vi "运维调试_五参数.vi"(11 "编号":string) -> ()   [LabVIEW 2016, in "斯坦道多参数.lvlib"]
uses:
  <vilib>/Utility/miscctls.llb/LVPointTypeDef.ctl
  <vilib>/Plasmionique/MB Master/MB_Master/MB_Master.lvclass
  <vilib>/ptbypt/NI_PtbyPt.lvlib
  <vilib>/Utility/config.llb/NI_LVConfig.lvlib
panel:
  in  "Serial Config":T1={"baud rate (bps)"=9600, "stop bits"=10, "parity"=0, "flow control"=0, "timeout"=2000, "retries"=1} {"stop bits" items=["1.0"=10, "1.5"=15, "2.0"=20]; "parity" items=["None", "Odd", "Even", "Mark", "Space"]; "flow control" items=["None", "XON/XOFF", "RTS/CTS", "XON/XOFF & RTS/CTS", "DTR/DSR", "XON/XOFF & DTR/DSR"]}
  in  "探头设置":bool
  in  "量程设置":bool
  out "显示框":T2={"显示控件"={"标题背景颜色"=3381759, "监测值背景颜色"=16777226, "监测参数"="", "状态1"="", "状态2"="", "数据标识"=""}, "显示控件 2"={"标题背景颜色"=3381759, "监测值背景颜色"=16777226, "监测参数"="", "状态1"="", "状态2"="", "数据标识"=""}, "显示控件 3"={"标题背景颜色"=3381759, "监测值背景颜色"=16777226, "监测参数"="", "状态1"="", "状态2"="", "数据标识"=""}, "显示控件 4"={"标题背景颜色"=3381759, "监测值背景颜色"=16777226, "监测参数"="", "状态1"="", "状态2"="", "数据标识"=""}, "显示控件 5"={"标题背景颜色"=3381759, "监测值背景颜色"=16777226, "监测参数"="", "状态1"="", "状态2"="", "数据标识"=""}, "显示控件 6"={"标题背景颜色"=3381759, "监测值背景颜色"=16777226, "监测参数"="", "状态1"="", "状态2"="", "数据标识"=""}, "显示控件 7"={"标题背景颜色"=3381759, "监测值背景颜色"=16777226, "监测参数"="", "状态1"="", "状态2"="", "数据标识"=""}, "显示控件 8"={"标题背景颜色"=3381759, "监测值背景颜色"=16777226, "监测参数"="", "状态1"="", "状态2"="", "数据标识"=""}, "显示控件 9"={"标题背景颜色"=3381759, "监测值背景颜色"=16777226, "监测参数"="", "状态1"="", "状态2"="", "数据标识"=""}, "显示控件 10"={"标题背景颜色"=3381759, "监测值背景颜色"=16777226, "监测参数"="", "状态1"="", "状态2"="", "数据标识"=""}}
  in  "传感器系列号":bool
  in  "水样保存组数":dbl caption="水样保存组数:"
  in  "水样稳定时间":dbl caption="水样稳定时间:"
  out "模块版本号":string
  out "权限等级":string
  in  "打开modbus":bool
  out "选项卡控件":enum32{"选项卡 1", "选项卡 2"}(tab)
  in  "VISA资源名称":refnum<visa-resource-name> caption="串口"
  in  "IP":string="localhost" caption="IP:"
  in  "Port":u16=502 caption="Port:"
  in  "自动断线重连":bool=TRUE
  in  "连接方式":u16(ring) items=["Modbus RTU", "Modbus TCP"]
  in  "密码锁":bool
  in  "设置页返回":bool
  in  "周期设置":bool
  out "当前串口":string
  out "运行状态":enum16{"空闲", "水样测试", "标样核查"}(ring)
  in  "停止":bool
  in  "标样核查":bool
  in  "水样测试":bool
  in  "设置":bool
  in  "探头校正返回":bool
  in  "探头校正":bool
  # "请设置仪器连接方式"
  # "组"
  # "min"
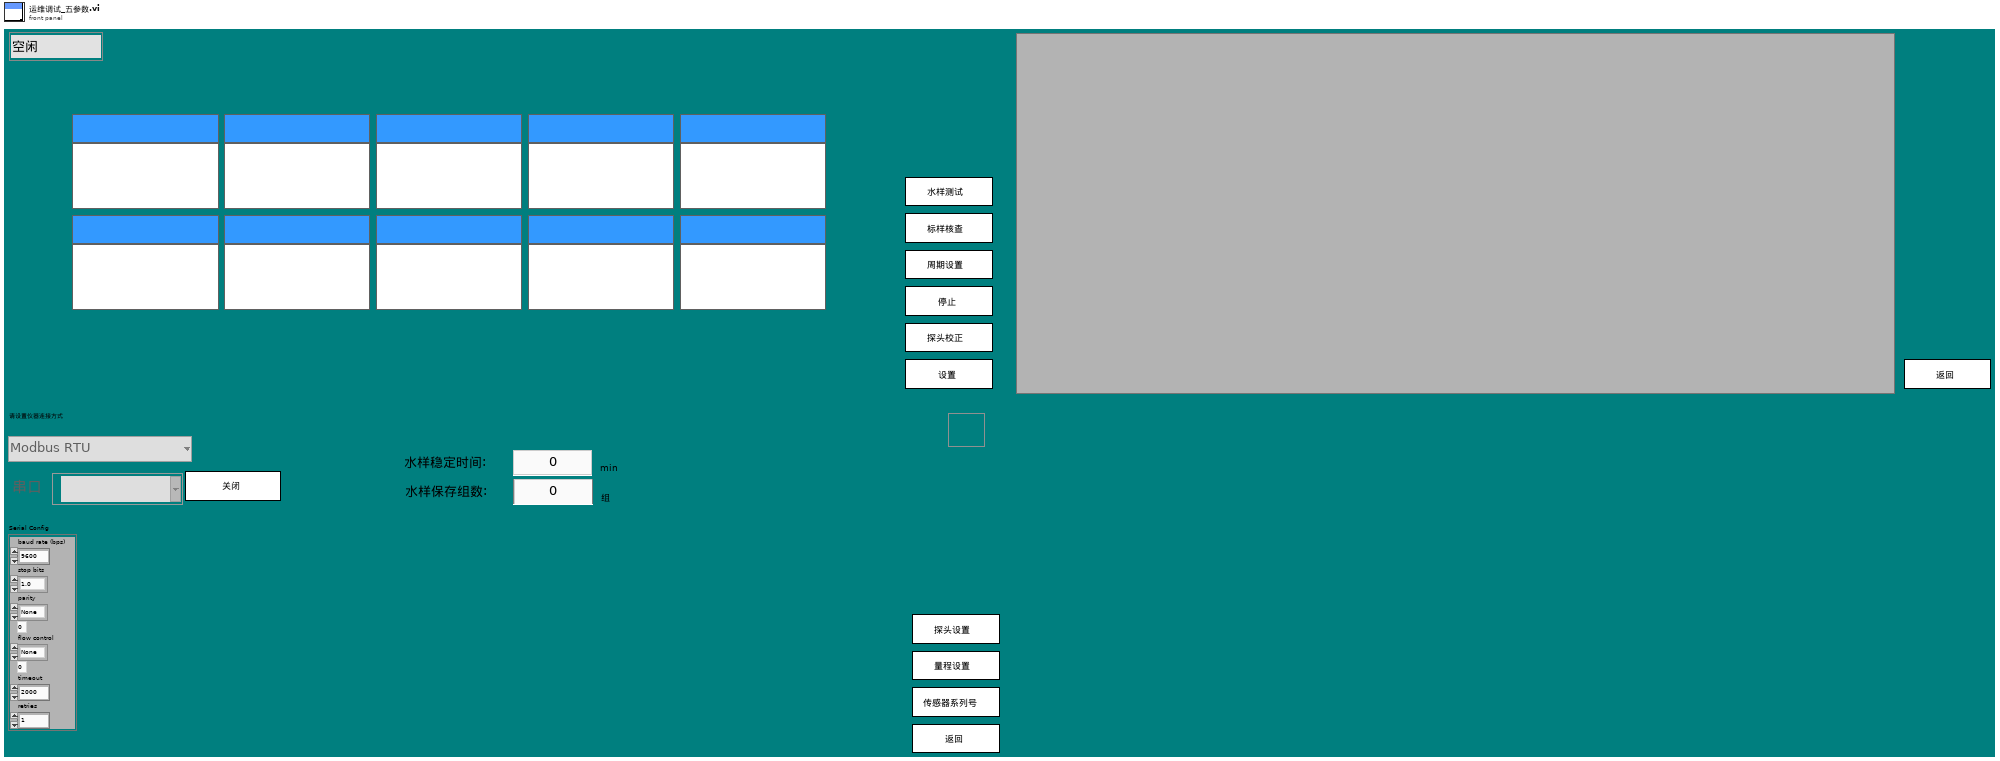
[diagram p1: front panel]
types:
  T1 = cluster{"baud rate (bps)":u32, "stop bits":u16, "parity":u16, "flow control":u16, "timeout":u32, "retries":i32}
  T2 = typedef "斯坦道多参数.lvlib/多状态显示框.ctl" = cluster{"显示控件":T3, "显示控件 2":T3, "显示控件 3":T3, "显示控件 4":T3, "显示控件 5":T3, "显示控件 6":T3, "显示控件 7":T3, "显示控件 8":T3, "显示控件 9":T3, "显示控件 10":T3}
  T3 = typedef "斯坦道多参数.lvlib/显示控件.ctl" = cluster{"标题背景颜色":u32, "监测值背景颜色":u32, "监测参数":string, "状态1":string, "状态2":string, "数据标识":string}
  T4 = typedef "斯坦道多参数.lvlib/数据流类型.ctl" = cluster{"cmd":enum16{"水样测试", "标样核查", "校准状态同步", "停止"}, "data":variant}
  T5 = typedef "LVPointTypeDef.ctl" = cluster{"Horizontal":i16, "Vertical":i16}
  T6 = enum8{"Enabled", "Disabled", "Disabled and Grayed Out"}
  T7 = cluster{"标签":string, "检测值1":cluster{"检测值":dbl, "单位":string, "启用":bool}, "检测值2":cluster{"检测值":dbl, "单位":string, "启用":bool}, "数据标识":string}[]
  T8 = cluster{"标签":string, "检测值1":cluster{"检测值":dbl, "单位":string, "启用":bool}, "检测值2":cluster{"检测值":dbl, "单位":string, "启用":bool}, "数据标识":string}
  T9 = cluster{"CH":u16, "监测值":dbl, "信号值":sgl, "数据标识":string}
  T10 = cluster{"温度测量值":sgl, "测量值":sgl, "温度偏移修正值":sgl, "信号值":sgl, "数据标识":string}
  T11 = cluster{"温度测量值":sgl, "DO%":sgl, "DOmg/L":sgl, "温度偏移修正值":sgl, "数据标识mg/L":string, "数据标识%":string}
  T12 = cluster{"周期设置类型":enum16{"定点启动", "间隔启动"}, "定时功能启用":bool, "定时间隔":u32, "24H周期设置":bool[], "延迟启动时间":u32}
  T13 = typedef "LVDateTimeRec.ctl" = cluster{"秒数的小数部分":dbl, "秒":i32, "分":i32, "时":i32, "日":i32, "月":i32, "年":i32, "天数（周）":i32, "天数（年）":i32, "DST":i32}
  T14 = cluster{"运行模式":enum16{"维护模式", "常规模式", "应急模式", "质控模式"}, "24H周期设置":bool[]}
  T15 = cluster{"Major":u16, "Minor":u16, "Fix":u16, "Build":u16}
  T16 = typedef "NI_LVConfig.lvlib/Config Data RefNum.ctl" = refnum<k1>
  T17 = enum32{"Bad", "Idle", "Run top level", "Running"}
  T18 = cluster{"ph":bool, "DO":bool, "Cond":bool, "Turb":bool, "叶绿素a":bool, "藻密度":bool, "ORP":bool, "cod":bool, "DO2":bool, "氯化物":bool, "氨氮":bool, "水中油":bool}
  T19 = cluster{"水温 (℃)":cluster{"量程下限":dbl, "量程上限":dbl}, "DO (mg/L)":cluster{"量程下限":dbl, "量程上限":dbl}, "DO (%)":cluster{"量程下限":dbl, "量程上限":dbl}, "pH":cluster{"量程下限":dbl, "量程上限":dbl}, "电导率 (μS/cm)":cluster{"量程下限":dbl, "量程上限":dbl}, "盐度":cluster{"量程下限":dbl, "量程上限":dbl}, "浊度 (NTU)":cluster{"量程下限":dbl, "量程上限":dbl}, "叶绿素a (μg/L)":cluster{"量程下限":dbl, "量程上限":dbl}, "藻密度 (cells/mL)":cluster{"量程下限":dbl, "量程上限":dbl}, "ORP (mV)":cluster{"量程下限":dbl, "量程上限":dbl}, "氯化物（mg/L）":cluster{"量程下限":dbl, "量程上限":dbl}, "COD":cluster{"量程下限":dbl, "量程上限":dbl}, "氨氮":cluster{"量程下限":dbl, "量程上限":dbl}, "水中油":cluster{"量程下限":dbl, "量程上限":dbl}}
  T20 = cluster{"周期设置类型":enum16{"定点启动", "间隔启动"}, "定时功能启用":bool, "定时间隔":u32, "24H周期设置":bool[], "延时启动时间":u32}
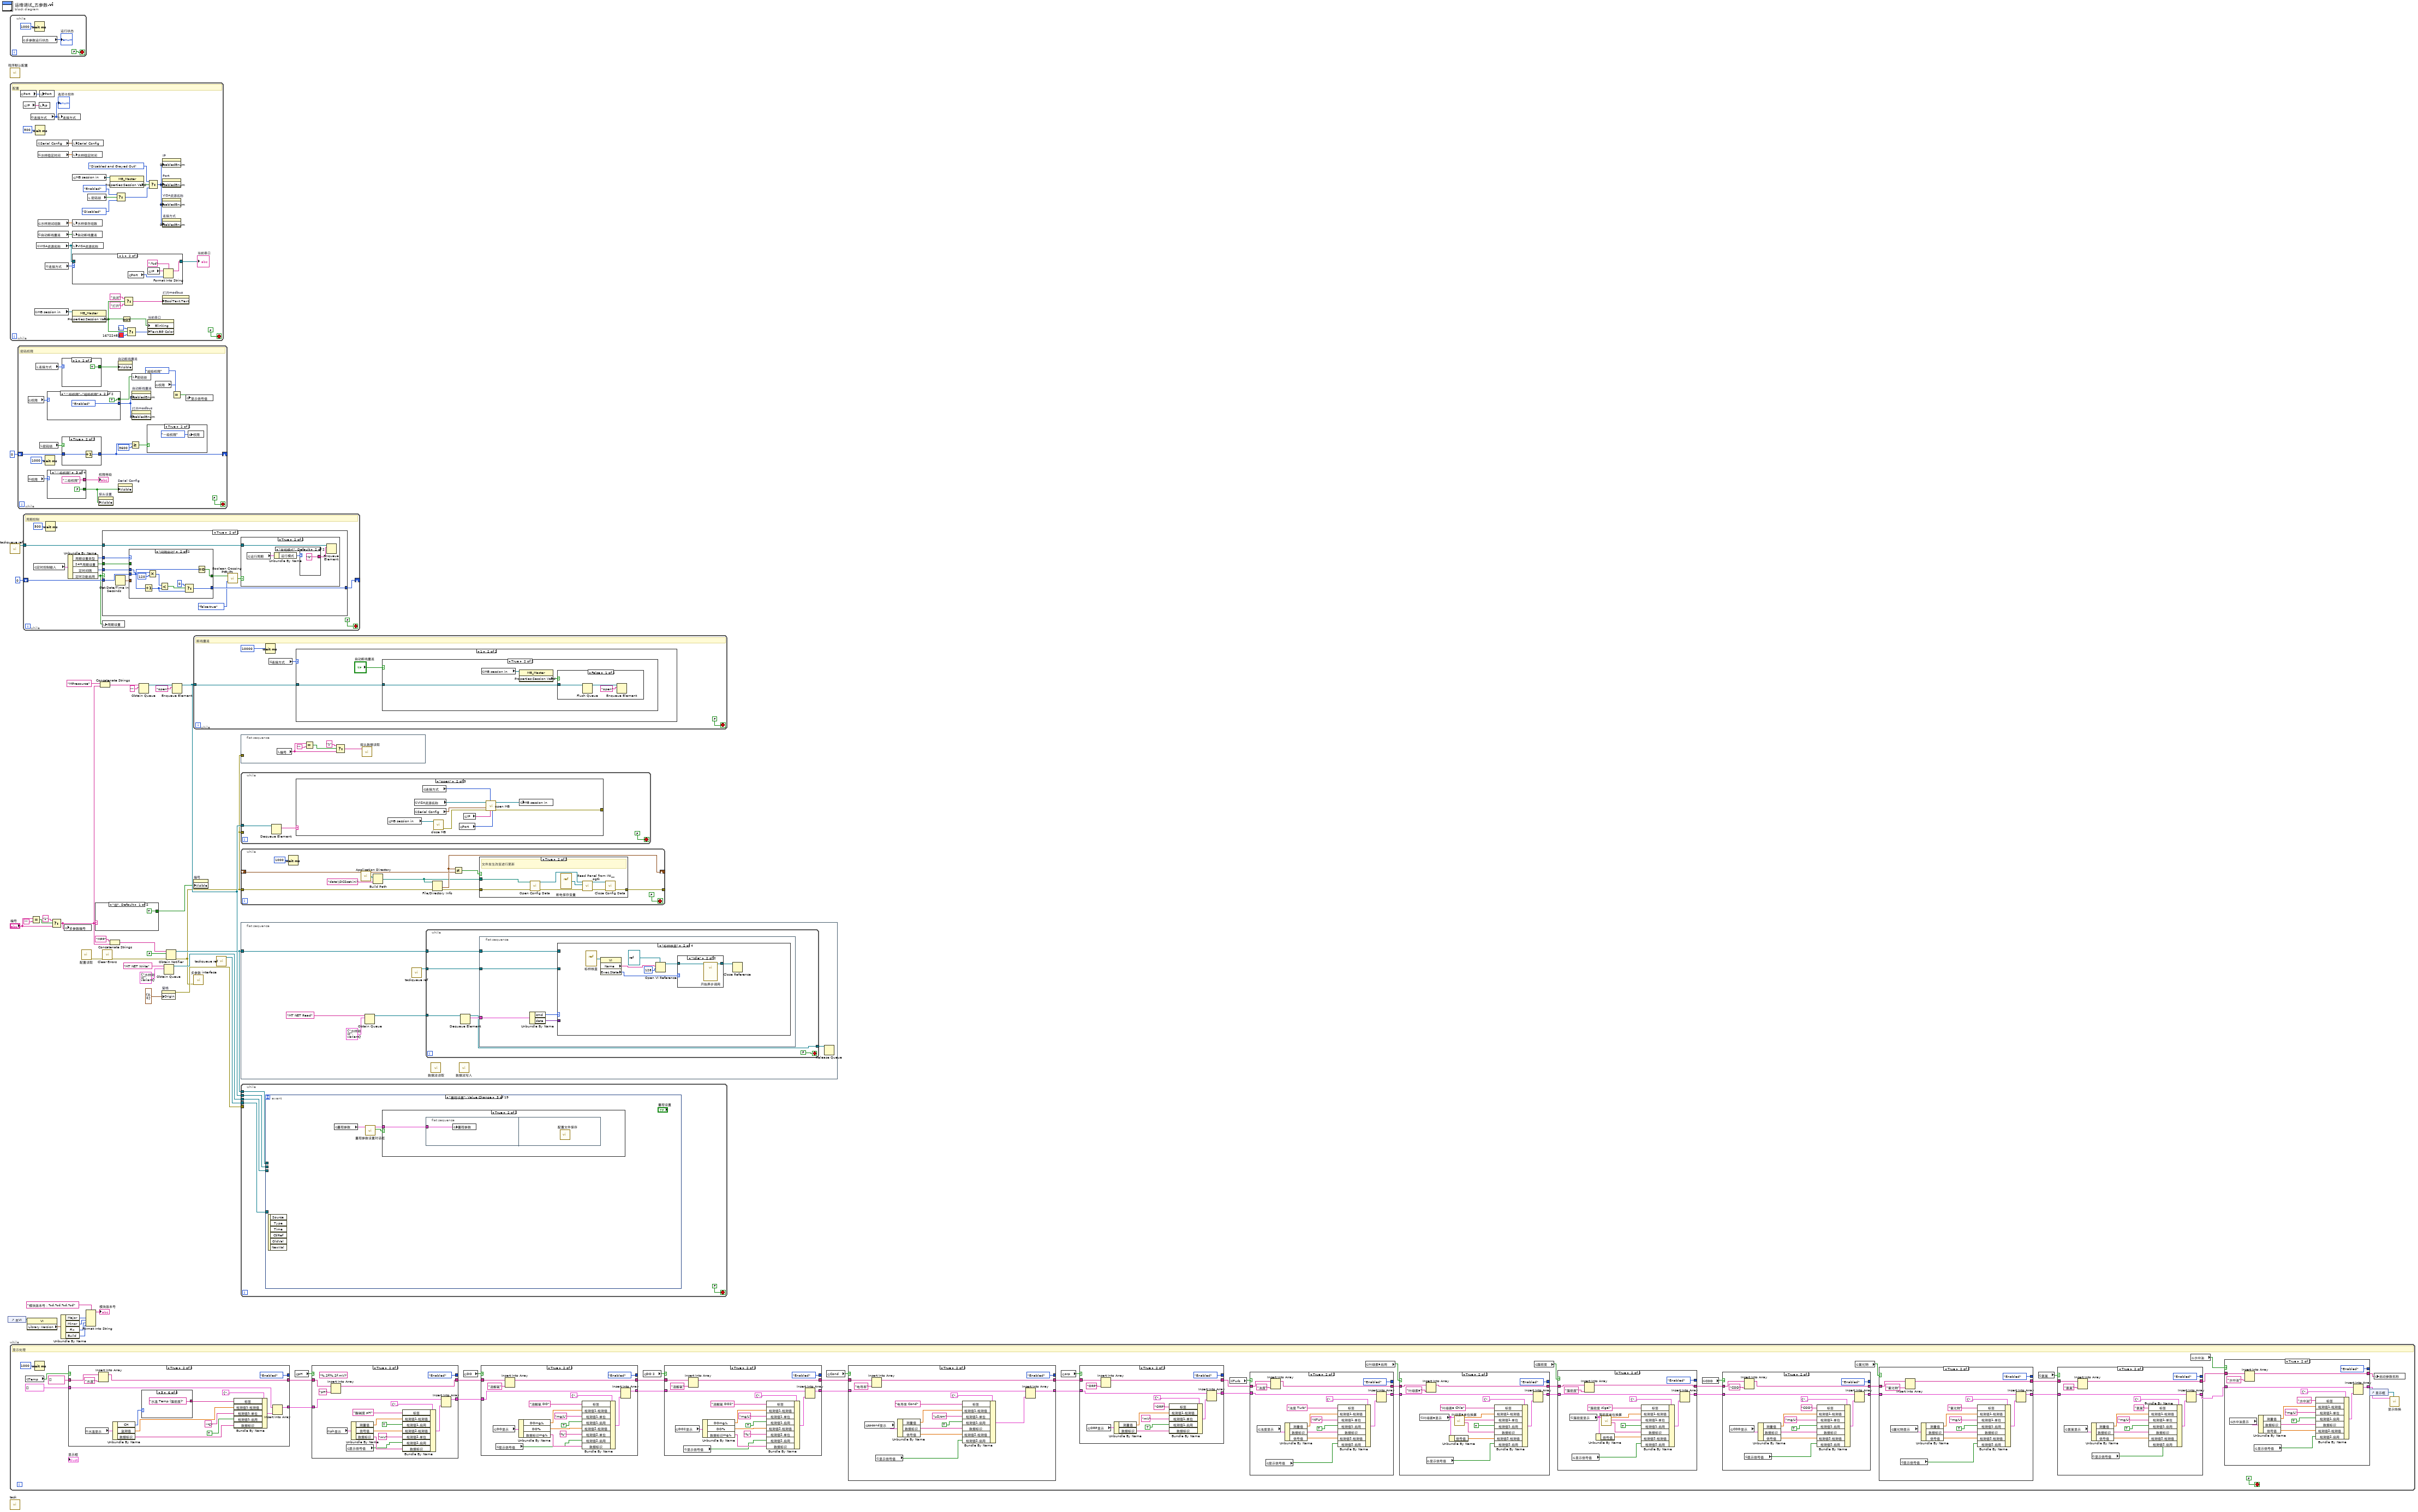
[diagram p0: block diagram]
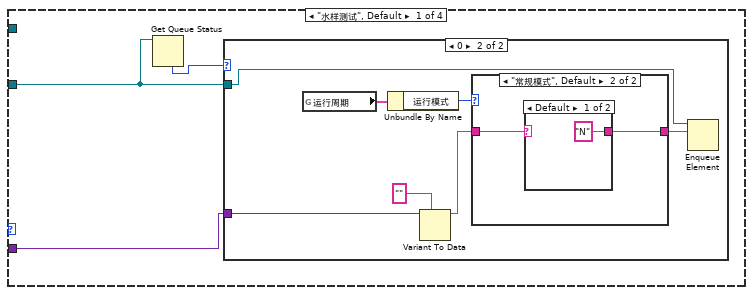
[diagram p2: hidden frame]
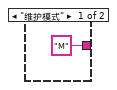
[diagram p4: hidden frame]
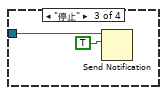
[diagram p7: hidden frame]
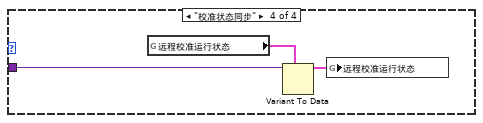
[diagram p8: hidden frame]
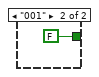
[diagram p9: hidden frame]
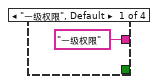
[diagram p17: hidden frame]
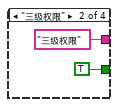
[diagram p18: hidden frame]
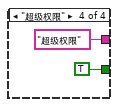
[diagram p19: hidden frame]
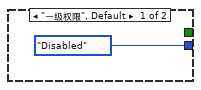
[diagram p20: hidden frame]
diagram:
  n1 = control-ref of="本VI"() -> (w22:refnum<vi>)
  n2 = while {
    stop <- FALSE stop-if-true
    n3 = global read "多参数全局变量.vi" "多参数运行状态"() -> (→"运行状态":u16)
    n4 = Wait (ms)(milliseconds to wait=u32 1000 ("等待时间（毫秒）")) -> ()  [unwired: 1 out]
  }
  n5 = call "程序默认配置.vi"() -> ()  [unwired: 11 in, 1 out]
  n6 = while {
    stop <- FALSE stop-if-true
    # "配置"
    n7 = global read "断电保存变量.vi" "Port"() -> (w55:u16)
    n8 = global read "断电保存变量.vi" "IP"() -> (w56:string)
    n9 = global read "断电保存变量.vi" "连接方式"() -> (w49:u16)
    "选项卡控件" <- w49
    n10 = global read "多参数全局变量.vi" "MB session in"() -> (w64:refnum<class "MB_Master.lvclass">)
    n11 = Wait (ms)(milliseconds to wait=u32 500 ("等待时间（毫秒）")) -> ()  [unwired: 1 out]
    n12 = global read "断电保存变量.vi" "VISA资源名称"() -> (w52:refnum<visa-resource-name>)
    n13 = global read "断电保存变量.vi" "Serial Config"() -> (w40:T1)
    n14 = global read "断电保存变量.vi" "水样稳定时间"() -> (w43:dbl)
    n15 = global read "断电保存变量.vi" "水样测试组数"() -> (w41:dbl)
    n16 = global read "断电保存变量.vi" "自动断线重连"() -> (w44:bool)
    n17 = local write "IP"(w56) -> ()
    n18 = local write "Port"(w55) -> ()
    n19 = global read "断电保存变量.vi" "连接方式"() -> (w53:u16)
    n20 = local write "连接方式"(w49) -> ()
    n21 = local write "Serial Config"(w40) -> ()
    n22 = local write "水样稳定时间"(w43) -> ()
    n23 = global read "多参数全局变量.vi" "MB session in"() -> (w67:refnum<class "MB_Master.lvclass">)
    n24 = local write "水样保存组数"(w41) -> ()
    n25 = local write "自动断线重连"(w44) -> ()
    n26 = local write "VISA资源名称"(w52) -> ()
    n27 = case shown="1" w53 {
      tunnel: w52 -> [w69 _]
      tunnel: [w69 w70] -> w51
      frame 0, Default {
      }
      frame 1 {
        n28 = global read "断电保存变量.vi" "Port"() -> (w71:u16)
        n29 = global read "断电保存变量.vi" "IP"() -> (w73:string)
        n30 = Format Into String(format string=":%d" ("格式字符串"), initial string=w73, w71) -> (resulting string=w70:string)  [unwired: 1 in, 1 out]
      }
    }
    "当前串口" <- w51
    n31 = property class="MB_Master"(reference=w64) -> ("Properties:Session Valid"=w48:bool)  [unwired: 1 in, 2 out]
    n32 = local read "密码锁"() -> (w60:bool)
    n33 = property class="MB_Master"(reference=w67) -> ("Properties:Session Valid"=w66:bool)  [unwired: 1 in, 2 out]
    n34 = Select(t=T6."Enabled" ("f"), s=w60, f=T6."Disabled") -> (s? t:f=w58:T6)
    n35 = Not(x=w48) -> (.not. x?=w50:bool)
    n36 = Select(t="关闭" ("布尔文本.文本"), s=w48, f="打开" ("布尔文本.文本")) -> (s? t:f=w61:string)
    n37 = Select(t=u32 16777216, s=w48, f=u32 16722483) -> (s? t:f=w45:u32)
    n38 = property on="当前串口" class="Str"("Blinking"=w50, "Text.BG Color"=w45) -> ()  [unwired: 2 in, 2 out]
    n39 = Select(t=T6."Disabled and Grayed Out" ("禁用"), s=w66, f=w58) -> (s? t:f=w54:T6)
    n40 = property on="IP" class="Str"("DisabledEnum"=w54) -> ()  [unwired: 2 in, 2 out]
    n41 = property on="Port" class="DigNum (strict)"("DisabledEnum"=w54) -> ()  [unwired: 2 in, 2 out]
    n42 = property on="VISA资源名称" class="VISAName"("DisabledEnum"=w54) -> ()  [unwired: 2 in, 2 out]
    n43 = property on="连接方式" class="Ring (strict)"("DisabledEnum"=w54) -> ()  [unwired: 2 in, 2 out]
    n44 = property on="打开modbus" class="Bool"("BoolText.Text"=w61) -> ()  [unwired: 2 in, 2 out]
  }
  n45 = call "taskqueue ref.vi"() -> ("队列输出"=w5:refnum<queue>)  [unwired: 10 in, 1 out]
  n46 = while {
    stop <- FALSE stop-if-true
    # "显示处理"
    n47 = global read "断电保存变量.vi" "Temp"() -> (w115:bool)
    n48 = Wait (ms)(milliseconds to wait=u32 1000 ("等待时间（毫秒）")) -> ()  [unwired: 1 out]
    n49 = case shown="True" w115 {
      tunnel: [w348 w360] -> w112
      tunnel: T7 [] ("数组") -> [w348 w361]
      tunnel: [T6."Disabled and Grayed Out" ("禁用") T6."Enabled" ("禁用")] -> _
      tunnel: string[] [] -> [w346 w351]
      tunnel: [w346 w350] -> w97
      frame False {
      }
      frame True {
        n50 = global read "多参数全局变量.vi" "水温显示"() -> (w358:T9)
        n51 = Insert Into Array(array=w351, new element="水温" ("新元素/子数组")) -> (w350:string[])  [unwired: 1 in]
        n52 = Unbundle By Name(w358) -> ("CH"=w357:u16, "监测值"=w355:dbl, "数据标识"=w354:string)
        n53 = case shown="5" w357 {
          tunnel: ["水温 Temp (pH)" ("监测参数1") "水温 Temp (DO)" ("监测参数1") "水温 Temp (浊度)" ("监测参数1") "水温 Temp (电导率)" ("监测参数1") "水温 Temp (叶绿素a)" ("监测参数1") "水温 Temp (藻密度)" ("监测参数1")] -> w363
          frame 0, Default {
          }
          frame 1 {
          }
          frame 2 {
          }
          frame 3 {
          }
          frame 4 {
          }
          frame 5 {
          }
        }
        n54 = Bundle By Name(cluster=T8 {"标签"="", "检测值1"={"检测值"=0.0, "单位"="", "启用"=FALSE}, "检测值2"={"检测值"=0.0, "单位"="", "启用"=FALSE}, "数据标识"=""} ("多参数状态显示"), "标签"=w363, "检测值1.检测值"=w355, "检测值1.单位"="℃", "检测值1.启用"=TRUE, "数据标识"=w354) -> (w362:T8)
        n55 = Insert Into Array(array=w361, new element=w362) -> (w360:T7)  [unwired: 1 in]
      }
    }
    n56 = global read "断电保存变量.vi" "pH"() -> (w113:bool)
    n57 = case shown="True" w113 {
      tunnel: [w329 w344] -> w110
      tunnel: w112 -> [w329 w345]
      tunnel: [T6."Disabled and Grayed Out" ("禁用") T6."Enabled" ("禁用")] -> _
      tunnel: w97 -> [w327 w333]
      tunnel: [w327 w332] -> w96
      frame False {
      }
      frame True {
        (unwired) "%.2f(%.2f mV)" ("格式字符串")
        n58 = global read "多参数全局变量.vi" "ph显示"() -> (w342:T10)
        n59 = Insert Into Array(array=w333, new element="pH" ("新元素/子数组")) -> (w332:string[])  [unwired: 1 in]
        n60 = global read "多参数全局变量.vi" "显示信号值"() -> (w330:bool)
        n61 = Unbundle By Name(w342) -> ("测量值"=w339:sgl, "信号值"=w337:sgl, "数据标识"=w335:string)
        n62 = Bundle By Name(cluster=T8 {"标签"="", "检测值1"={"检测值"=0.0, "单位"="", "启用"=FALSE}, "检测值2"={"检测值"=0.0, "单位"="", "启用"=FALSE}, "数据标识"=""} ("多参数状态显示"), "标签"="酸碱度 pH" ("监测参数2"), "检测值1.检测值"=w339, "检测值1.启用"=TRUE, "检测值2.检测值"=w337, "检测值2.单位"="mV", "检测值2.启用"=w330, "数据标识"=w335) -> (w334:T8)
        n63 = Insert Into Array(array=w345, new element=w334) -> (w344:T7)  [unwired: 1 in]
      }
    }
    n64 = global read "断电保存变量.vi" "DO"() -> (w111:bool)
    n65 = case shown="True" w111 {
      tunnel: [w309 w325] -> w89
      tunnel: w110 -> [w309 w326]
      tunnel: [T6."Disabled and Grayed Out" ("禁用") T6."Enabled" ("禁用")] -> _
      tunnel: w96 -> [w307 w313]
      tunnel: [w307 w312] -> w88
      frame False {
      }
      frame True {
        n66 = global read "多参数全局变量.vi" "DO显示"() -> (w323:T11)
        n67 = global read "多参数全局变量.vi" "显示信号值"() -> (w310:bool)
        n68 = Insert Into Array(array=w313, new element="溶解氧" ("新元素/子数组")) -> (w312:string[])  [unwired: 1 in]
        n69 = Unbundle By Name(w323) -> ("DOmg/L"=w320:sgl, "DO%"=w318:sgl, "数据标识mg/L"=w317:string)
        n70 = Bundle By Name(cluster=T8 {"标签"="", "检测值1"={"检测值"=0.0, "单位"="", "启用"=FALSE}, "检测值2"={"检测值"=0.0, "单位"="", "启用"=FALSE}, "数据标识"=""} ("多参数状态显示"), "标签"="溶解氧 DO" ("监测参数2"), "检测值1.检测值"=w320, "检测值1.单位"="mg/L", "检测值1.启用"=TRUE, "检测值2.检测值"=w318, "检测值2.单位"="%", "检测值2.启用"=w310, "数据标识"=w317) -> (w314:T8)
        n71 = Insert Into Array(array=w326, new element=w314) -> (w325:T7)  [unwired: 1 in]
      }
    }
    n72 = global read "断电保存变量.vi" "DO 2"() -> (w90:bool)
    n73 = case shown="True" w90 {
      tunnel: [w177 w193] -> w87
      tunnel: w89 -> [w177 w194]
      tunnel: [T6."Disabled and Grayed Out" ("禁用") T6."Enabled" ("禁用")] -> _
      tunnel: w88 -> [w175 w181]
      tunnel: [w175 w180] -> w86
      frame False {
      }
      frame True {
        n74 = global read "多参数全局变量.vi" "DO2显示"() -> (w191:T11)
        n75 = global read "多参数全局变量.vi" "显示信号值"() -> (w178:bool)
        n76 = Insert Into Array(array=w181, new element="溶解氧" ("新元素/子数组")) -> (w180:string[])  [unwired: 1 in]
        n77 = Unbundle By Name(w191) -> ("DOmg/L"=w188:sgl, "DO%"=w186:sgl, "数据标识mg/L"=w185:string)
        n78 = Bundle By Name(cluster=T8 {"标签"="", "检测值1"={"检测值"=0.0, "单位"="", "启用"=FALSE}, "检测值2"={"检测值"=0.0, "单位"="", "启用"=FALSE}, "数据标识"=""} ("多参数状态显示"), "标签"="溶解氧 DO2" ("监测参数2"), "检测值1.检测值"=w188, "检测值1.单位"="mg/L", "检测值1.启用"=TRUE, "检测值2.检测值"=w186, "检测值2.单位"="%", "检测值2.启用"=w178, "数据标识"=w185) -> (w182:T8)
        n79 = Insert Into Array(array=w194, new element=w182) -> (w193:T7)  [unwired: 1 in]
      }
    }
    n80 = global read "断电保存变量.vi" "Cond"() -> (w109:bool)
    n81 = case shown="True" w109 {
      tunnel: w87 -> [w290 w306]
      tunnel: [w290 w292] -> w101
      tunnel: [T6."Disabled and Grayed Out" ("禁用") T6."Enabled" ("禁用")] -> _
      tunnel: w86 -> [w288 w296]
      tunnel: [w288 w295] -> w95
      frame False {
      }
      frame True {
        n82 = global read "多参数全局变量.vi" "spcond显示"() -> (w304:T10)
        n83 = Insert Into Array(array=w296, new element="电导率" ("新元素/子数组")) -> (w295:string[])  [unwired: 1 in]
        n84 = global read "多参数全局变量.vi" "显示信号值"() -> (w291:bool)
        n85 = Unbundle By Name(w304) -> ("测量值"=w300:sgl, "数据标识"=w298:string, "信号值"=w293:sgl)
        n86 = Bundle By Name(cluster=T8 {"标签"="", "检测值1"={"检测值"=0.0, "单位"="", "启用"=FALSE}, "检测值2"={"检测值"=0.0, "单位"="", "启用"=FALSE}, "数据标识"=""} ("多参数状态显示"), "标签"="电导率 Cond" ("监测参数2"), "检测值1.检测值"=w300, "检测值1.单位"="μS/cm", "检测值1.启用"=TRUE, "数据标识"=w298, "检测值2.检测值"=w293, "检测值2.启用"=w291) -> (w297:T8)
        n87 = Insert Into Array(array=w306, new element=w297) -> (w292:T7)  [unwired: 1 in]
      }
    }
    n88 = global read "断电保存变量.vi" "orp"() -> (w103:bool)
    n89 = case shown="True" w103 {
      tunnel: w101 -> [w216 w230]
      tunnel: [w216 w229] -> w102
      tunnel: [T6."Disabled and Grayed Out" ("禁用") T6."Enabled" ("禁用")] -> _
      tunnel: w95 -> [w214 w219]
      tunnel: [w214 w218] -> w94
      frame False {
      }
      frame True {
        n90 = global read "多参数全局变量.vi" "ORP显示"() -> (w227:T10)
        n91 = Insert Into Array(array=w219, new element="ORP" ("新元素/子数组")) -> (w218:string[])  [unwired: 1 in]
        n92 = Unbundle By Name(w227) -> ("测量值"=w222:sgl, "数据标识"=w221:string)
        n93 = Bundle By Name(cluster=T8 {"标签"="", "检测值1"={"检测值"=0.0, "单位"="", "启用"=FALSE}, "检测值2"={"检测值"=0.0, "单位"="", "启用"=FALSE}, "数据标识"=""} ("多参数状态显示"), "标签"="ORP" ("监测参数2"), "检测值1.检测值"=w222, "检测值1.单位"="mV", "检测值1.启用"=TRUE, "数据标识"=w221) -> (w220:T8)
        n94 = Insert Into Array(array=w230, new element=w220) -> (w229:T7)  [unwired: 1 in]
      }
    }
    n95 = global read "断电保存变量.vi" "Turb"() -> (w108:bool)
    n96 = case shown="True" w108 {
      tunnel: w102 -> [w271 w287]
      tunnel: [w271 w286] -> w107
      tunnel: [T6."Disabled and Grayed Out" ("禁用") T6."Enabled" ("禁用")] -> _
      tunnel: w94 -> [w269 w276]
      tunnel: [w269 w275] -> w93
      frame False {
      }
      frame True {
        n97 = global read "多参数全局变量.vi" "浊度显示"() -> (w284:T10)
        n98 = global read "多参数全局变量.vi" "显示信号值"() -> (w272:bool)
        n99 = Insert Into Array(array=w276, new element="浊度" ("新元素/子数组")) -> (w275:string[])  [unwired: 1 in]
        n100 = Unbundle By Name(w284) -> ("测量值"=w279:sgl, "数据标识"=w278:string, "信号值"=w273:sgl)
        n101 = Bundle By Name(cluster=T8 {"标签"="", "检测值1"={"检测值"=0.0, "单位"="", "启用"=FALSE}, "检测值2"={"检测值"=0.0, "单位"="", "启用"=FALSE}, "数据标识"=""} ("多参数状态显示"), "标签"="浊度 Turb" ("监测参数2"), "检测值1.检测值"=w279, "检测值1.单位"="NTU", "检测值1.启用"=TRUE, "数据标识"=w278, "检测值2.检测值"=w273, "检测值2.启用"=w272) -> (w277:T8)
        n102 = Insert Into Array(array=w287, new element=w277) -> (w286:T7)  [unwired: 1 in]
      }
    }
    n103 = global read "断电保存变量.vi" "叶绿素a启用"() -> (w106:bool)
    n104 = case shown="True" w106 {
      tunnel: w107 -> [w252 w268]
      tunnel: [w252 w267] -> w104
      tunnel: [T6."Disabled and Grayed Out" ("禁用") T6."Enabled" ("禁用")] -> _
      tunnel: w93 -> [w250 w261]
      tunnel: [w250 w260] -> w92
      frame False {
      }
      frame True {
        n105 = global read "多参数全局变量.vi" "叶绿素a显示"() -> (w255:T10)
        n106 = Insert Into Array(array=w261, new element="叶绿素a" ("新元素/子数组")) -> (w260:string[])  [unwired: 1 in]
        n107 = global read "多参数全局变量.vi" "显示信号值"() -> (w253:bool)
        n108 = Unbundle By Name(w255) -> ("信号值"=w254:sgl)
        n109 = call "叶绿素a单位换算.vi"("叶绿素a显示"=w255) -> ("数据标识"=w256:string, "检测值1.单位"=w258:string, "测量值"=w257:sgl)  [unwired: 8 in]
        n110 = Bundle By Name(cluster=T8 {"标签"="", "检测值1"={"检测值"=0.0, "单位"="", "启用"=FALSE}, "检测值2"={"检测值"=0.0, "单位"="", "启用"=FALSE}, "数据标识"=""} ("多参数状态显示"), "标签"="叶绿素a Chla" ("监测参数2"), "检测值1.检测值"=w257, "检测值1.单位"=w258, "检测值1.启用"=TRUE, "数据标识"=w256, "检测值2.检测值"=w254, "检测值2.启用"=w253) -> (w262:T8)
        n111 = Insert Into Array(array=w268, new element=w262) -> (w267:T7)  [unwired: 1 in]
      }
    }
    n112 = global read "断电保存变量.vi" "藻密度"() -> (w105:bool)
    n113 = case shown="True" w105 {
      tunnel: w104 -> [w233 w249]
      tunnel: [w233 w248] -> w100
      tunnel: [T6."Disabled and Grayed Out" ("禁用") T6."Enabled" ("禁用")] -> _
      tunnel: w92 -> [w231 w242]
      tunnel: [w231 w241] -> w91
      frame False {
      }
      frame True {
        n114 = global read "多参数全局变量.vi" "藻密度显示"() -> (w236:T10)
        n115 = global read "多参数全局变量.vi" "显示信号值"() -> (w234:bool)
        n116 = Insert Into Array(array=w242, new element="藻密度" ("新元素/子数组")) -> (w241:string[])  [unwired: 1 in]
        n117 = Unbundle By Name(w236) -> ("信号值"=w235:sgl)
        n118 = call "藻密度单位换算.vi"("藻密度显示"=w236) -> ("数据标识"=w238:string, "检测值1.单位"=w237:string, "测量值"=w239:sgl)  [unwired: 8 in]
        n119 = Bundle By Name(cluster=T8 {"标签"="", "检测值1"={"检测值"=0.0, "单位"="", "启用"=FALSE}, "检测值2"={"检测值"=0.0, "单位"="", "启用"=FALSE}, "数据标识"=""} ("多参数状态显示"), "标签"="藻密度 Algal" ("监测参数2"), "检测值1.检测值"=w239, "检测值1.单位"=w237, "检测值1.启用"=TRUE, "数据标识"=w238, "检测值2.检测值"=w235, "检测值2.启用"=w234) -> (w243:T8)
        n120 = Insert Into Array(array=w249, new element=w243) -> (w248:T7)  [unwired: 1 in]
      }
    }
    n121 = global read "断电保存变量.vi" "COD"() -> (w99:bool)
    n122 = case shown="True" w99 {
      tunnel: w100 -> [w197 w213]
      tunnel: [w197 w212] -> w82
      tunnel: [T6."Disabled and Grayed Out" ("禁用") T6."Enabled" ("禁用")] -> _
      tunnel: w91 -> [w195 w202]
      tunnel: [w195 w201] -> w83
      frame False {
      }
      frame True {
        n123 = global read "多参数全局变量.vi" "COD显示"() -> (w210:T10)
        n124 = Insert Into Array(array=w202, new element="COD" ("新元素/子数组")) -> (w201:string[])  [unwired: 1 in]
        n125 = global read "多参数全局变量.vi" "显示信号值"() -> (w198:bool)
        n126 = Unbundle By Name(w210) -> ("测量值"=w205:sgl, "数据标识"=w204:string, "信号值"=w199:sgl)
        n127 = Bundle By Name(cluster=T8 {"标签"="", "检测值1"={"检测值"=0.0, "单位"="", "启用"=FALSE}, "检测值2"={"检测值"=0.0, "单位"="", "启用"=FALSE}, "数据标识"=""} ("多参数状态显示"), "标签"="COD" ("监测参数2"), "检测值1.检测值"=w205, "检测值1.单位"="mg/L", "检测值1.启用"=TRUE, "数据标识"=w204, "检测值2.检测值"=w199, "检测值2.启用"=w198) -> (w203:T8)
        n128 = Insert Into Array(array=w213, new element=w203) -> (w212:T7)  [unwired: 1 in]
      }
    }
    n129 = global read "断电保存变量.vi" "氯化物"() -> (w84:bool)
    n130 = case shown="True" w84 {
      tunnel: w82 -> [w158 w174]
      tunnel: [w158 w173] -> w80
      tunnel: [T6."Disabled and Grayed Out" ("禁用") T6."Enabled" ("禁用")] -> _
      tunnel: w83 -> [w156 w163]
      tunnel: [w156 w162] -> w81
      frame False {
      }
      frame True {
        n131 = global read "多参数全局变量.vi" "氯化物显示"() -> (w171:T10)
        n132 = global read "多参数全局变量.vi" "显示信号值"() -> (w159:bool)
        n133 = Insert Into Array(array=w163, new element="氯化物" ("新元素/子数组")) -> (w162:string[])  [unwired: 1 in]
        n134 = Unbundle By Name(w171) -> ("测量值"=w166:sgl, "数据标识"=w165:string, "信号值"=w160:sgl)
        n135 = Bundle By Name(cluster=T8 {"标签"="", "检测值1"={"检测值"=0.0, "单位"="", "启用"=FALSE}, "检测值2"={"检测值"=0.0, "单位"="", "启用"=FALSE}, "数据标识"=""} ("多参数状态显示"), "标签"="氯化物" ("监测参数2"), "检测值1.检测值"=w166, "检测值1.单位"="mg/L", "检测值1.启用"=TRUE, "数据标识"=w165, "检测值2.检测值"=w160, "检测值2.启用"=w159) -> (w164:T8)
        n136 = Insert Into Array(array=w174, new element=w164) -> (w173:T7)  [unwired: 1 in]
      }
    }
    n137 = global read "断电保存变量.vi" "氨氮"() -> (w79:bool)
    n138 = case shown="True" w79 {
      tunnel: w80 -> [w139 w155]
      tunnel: [w139 w154] -> w77
      tunnel: [T6."Disabled and Grayed Out" ("禁用") T6."Enabled" ("禁用")] -> _
      tunnel: w81 -> [w137 w144]
      tunnel: [w137 w143] -> w78
      frame False {
      }
      frame True {
        n139 = global read "多参数全局变量.vi" "氨氮显示"() -> (w152:T10)
        n140 = Insert Into Array(array=w144, new element="氨氮" ("新元素/子数组")) -> (w143:string[])  [unwired: 1 in]
        n141 = Unbundle By Name(w152) -> ("测量值"=w147:sgl, "数据标识"=w146:string, "信号值"=w141:sgl)
        n142 = global read "多参数全局变量.vi" "显示信号值"() -> (w140:bool)
        n143 = Bundle By Name(cluster=T8 {"标签"="", "检测值1"={"检测值"=0.0, "单位"="", "启用"=FALSE}, "检测值2"={"检测值"=0.0, "单位"="", "启用"=FALSE}, "数据标识"=""} ("多参数状态显示"), "标签"="氨氮" ("监测参数2"), "检测值1.检测值"=w147, "检测值1.单位"="mg/L", "检测值1.启用"=TRUE, "数据标识"=w146, "检测值2.检测值"=w141, "检测值2.启用"=w140) -> (w145:T8)
        n144 = Insert Into Array(array=w155, new element=w145) -> (w154:T7)  [unwired: 1 in]
      }
    }
    n145 = global read "断电保存变量.vi" "水中油"() -> (w75:bool)
    n146 = case shown="True" w75 {
      tunnel: w77 -> [w120 w136]
      tunnel: [w120 w135] -> w76
      tunnel: [T6."Disabled and Grayed Out" ("禁用") T6."Enabled" ("禁用")] -> _
      tunnel: w78 -> [w118 w125]
      tunnel: [w118 w124] -> w74
      frame False {
      }
      frame True {
        n147 = global read "多参数全局变量.vi" "水中油显示"() -> (w133:T10)
        n148 = Insert Into Array(array=w125, new element="水中油" ("新元素/子数组")) -> (w124:string[])  [unwired: 1 in]
        n149 = global read "多参数全局变量.vi" "显示信号值"() -> (w121:bool)
        n150 = Unbundle By Name(w133) -> ("测量值"=w128:sgl, "数据标识"=w127:string, "信号值"=w122:sgl)
        n151 = Bundle By Name(cluster=T8 {"标签"="", "检测值1"={"检测值"=0.0, "单位"="", "启用"=FALSE}, "检测值2"={"检测值"=0.0, "单位"="", "启用"=FALSE}, "数据标识"=""} ("多参数状态显示"), "标签"="水中油" ("监测参数2"), "检测值1.检测值"=w128, "检测值1.单位"="mg/L", "检测值1.启用"=TRUE, "数据标识"=w127, "检测值2.检测值"=w122, "检测值2.启用"=w121) -> (w126:T8)
        n152 = Insert Into Array(array=w136, new element=w126) -> (w135:T7)  [unwired: 1 in]
      }
    }
    n153 = control-ref of="显示框"() -> (w85:refnum<vi>)
    n154 = global write "多参数全局变量.vi" "启动参数名称"(w74) -> ()
    n155 = call "显示转换.vi"("显示控件"=w85, "数组输入"=w76) -> ()  [unwired: 10 in]
  }
  n156 = call "task.vi"() -> ()  [unwired: 12 in]
  n157 = while {
    shift-right: [w383] -> _
    shift-left: u32 0 ("等待时间（毫秒）") -> [w384]
    stop <- FALSE stop-if-true
    # "密码权限"
    n158 = global read "多参数全局变量.vi" "权限"() -> (w375:enum16{"一级权限", "二级权限", "三级权限", "超级权限"})
    n159 = global read "多参数全局变量.vi" "权限"() -> (w376:enum16{"一级权限", "二级权限", "三级权限", "超级权限"})
    n160 = local read "连接方式"() -> (w380:u16)
    n161 = local read "密码锁"() -> (w385:bool)
    n162 = Wait (ms)(milliseconds to wait=u32 1000 ("等待时间（毫秒）")) -> ()  [unwired: 1 out]
    n163 = case shown="\"二级权限\"..\"超级权限\"" w375 {
      tunnel: [T6."Disabled" ("禁用") T6."Enabled" ("禁用")] -> w378
      tunnel: [_ TRUE ("可见")] -> w374
      frame "一级权限", Default {
      }
      frame "二级权限".."超级权限" {
      }
    }
    n164 = case shown="\"二级权限\"" w376 {
      tunnel: ["一级权限" ("权限等级") "三级权限" ("权限等级") "二级权限" ("权限等级") "超级权限" ("权限等级")] -> w377
      tunnel: [_ TRUE FALSE TRUE] -> w373
      frame "一级权限", Default {
      }
      frame "三级权限" {
      }
      frame "二级权限" {
      }
      frame "超级权限" {
      }
    }
    "权限等级" <- w377
    n165 = case shown="1" w380 {
      tunnel: [_ TRUE ("可见")] -> w379
      frame 0, Default {
      }
      frame 1 {
      }
    }
    n166 = case shown="True" w385 {
      tunnel: w384 -> [_ w391]
      tunnel: [_ w390] -> w383
      frame False {
      }
      frame True {
        n167 = Increment(x=w391) -> (x+1=w390:u32)
      }
    }
    n168 = property on="探头设置" class="Bool"("Visible"=w373) -> ()  [unwired: 2 in, 2 out]
    n169 = property on="自动断线重连" class="Bool (strict)"("Visible"=w379) -> ()  [unwired: 2 in, 2 out]
    n170 = property on="Serial Config" class="Clust (strict)"("Visible"=w373) -> ()  [unwired: 2 in, 2 out]
    n171 = Greater Or Equal?(x=w383, y=u32 3600) -> (x >= y?=w381:bool)
    n172 = local write "密码锁"(w374) -> ()
    n173 = property on="自动断线重连" class="Bool (strict)"("DisabledEnum"=w378) -> ()  [unwired: 2 in, 2 out]
    n174 = property on="打开modbus" class="Bool"("DisabledEnum"=w378) -> ()  [unwired: 2 in, 2 out]
    n175 = case shown="True" w381 {
      frame False {
      }
      frame True {
        n176 = global write "多参数全局变量.vi" "权限"(enum16{"一级权限", "二级权限", "三级权限", "超级权限"}."一级权限" ("权限")) -> ()
      }
    }
    n177 = global read "多参数全局变量.vi" "权限"() -> (w372:enum16{"一级权限", "二级权限", "三级权限", "超级权限"})
    n178 = Equal?(x=w372, y=enum16{"一级权限", "二级权限", "三级权限", "超级权限"}."超级权限") -> (x = y?=w371:bool)
    n179 = global write "多参数全局变量.vi" "显示信号值"(w371) -> ()
  }
  n180 = while {
    shift-right: [w404] -> _
    shift-left: u32 0 ("等待时间（毫秒）") -> [w405]
    tunnel: w5 -> [w402]
    stop <- FALSE stop-if-true
    # "周期控制"
    n181 = global read "断电保存变量.vi" "定时控制输入"() -> (w407:T12)
    n182 = Wait (ms)(milliseconds to wait=u32 500 ("等待时间（毫秒）")) -> ()  [unwired: 1 out]
    n183 = Unbundle By Name(w407) -> ("周期设置类型"=w409:enum16{"定点启动", "间隔启动"}, "24H周期设置"=w408:bool[], "定时间隔"=w406:u32, "定时功能启用"=w403:bool)
    n184 = case shown="True" w403 {
      tunnel: w409 -> [_ w420]
      tunnel: w408 -> [_ w419]
      tunnel: w406 -> [_ w418]
      tunnel: w405 -> [_ w417]
      tunnel: [_ w416] -> w404
      tunnel: w402 -> [_ w415]
      frame False {
      }
      frame True {
        n185 = Get Date/Time In Seconds() -> (seconds since 1Jan1904=w421:timestamp)
        n186 = case shown="\"间隔启动\"" w420 {
          tunnel: w421 -> [w437 _]
          tunnel: w419 -> [w434 _]
          tunnel: [w428 w445] -> w414
          tunnel: w418 -> [_ w444]
          tunnel: w417 -> [_ w446]
          tunnel: [_ w440] -> w416
          frame "定点启动", Default {
            n187 = Seconds To Date/Time(time stamp (now)=w437) -> (date time rec=w436:T13)  [unwired: 1 in]
            n188 = Unbundle By Name(w436) -> ("时"=w435:i32, "分"=w433:i32, "秒"=w432:i32)
            n189 = Index Array(array=w434, index=w435) -> (element=w431:bool)
            n190 = Equal To 0?(x=w433) -> (x = 0?=w430:bool)
            n191 = Equal To 0?(x=w432) -> (x = 0?=w429:bool)
            n192 = Compound Arithmetic op=AND ("复合运算")(w431, w430, w429) -> (w428:bool)
          }
          frame "间隔启动" {
            n193 = Increment(x=w446) -> (x+1=w439:u32)
            n194 = Multiply(x=w444, y=u32 120) -> (x*y=w438:u32)
            n195 = Less?(x=w438, y=w439) -> (x < y?=w442:bool)
            n196 = Select(t=u32 0 ("y"), s=w442, f=w439) -> (s? t:f=w440:u32)
            n197 = Equal To 0?(x=w446) -> (x = 0?=w445:bool)
          }
        }
        n198 = call <vilib>:"Boolean Crossing PtByPt.vi"("direction"=enum16{"either", "false-true", "true-false"}."false-true", "input"=w414) -> ("crossing"=w413:bool)  [unwired: 1 in]
        n199 = case shown="True" w413 {
          tunnel: w415 -> [_ w423]
          frame False {
          }
          frame True {
            n200 = global read "断电保存变量.vi" "运行周期"() -> (w424:T14)
            n201 = Unbundle By Name(w424) -> ("运行模式"=w425:enum16{"维护模式", "常规模式", "应急模式", "质控模式"})
            n202 = case shown="\"常规模式\", Default" w425 {
              tunnel: ["M" ("数据标记表") "N" ("数据标记表")] -> w422
              frame "维护模式" {
              }
              frame "常规模式", Default {
              }
            }
            n203 = Enqueue Element(queue=w423, element=w422) -> ()  [unwired: 2 in, 3 out]
          }
        }
      }
    }
    n204 = local write "周期设置"(w403) -> ()
  }
  n205 = property class="VI"(reference=w22) -> ("Library.Version"=w21:T15)  [unwired: 1 in, 2 out]
  n206 = Equal?(x="编号", y="") -> (x = y?=w13:bool)
  n207 = Select(t="1", s=w13, f="编号") -> (s? t:f=w11:string)
  n208 = Unbundle By Name(w21) -> ("Major"=w19:u16, "Minor"=w18:u16, "Fix"=w17:u16, "Build"=w16:u16)
  n209 = global write "多参数全局变量.vi" "多参数编号"(w11) -> ()
  n210 = call "配置读取.vi"() -> ("error out"=w2:errorcluster)  [unwired: 11 in]
  n211 = Format Into String(format string="模块版本号：%d.%d.%d.%d" ("格式字符串"), w19, w18, w17, w16) -> (resulting string=→"模块版本号":string)  [unwired: 2 in, 1 out]
  n212 = case shown="\"假\", Default" w11 {
    tunnel: [TRUE ("可见") FALSE ("可见")] -> w23
    frame "假", Default {
    }
    frame "001" {
    }
  }
  n213 = Concatenate Strings("MPresource" ("名称（未命名）"), w11) -> (w29:string)
  n214 = call <vilib>:"Clear Errors.vi"("error in (no error)"=w2) -> ("error out"=w1:errorcluster)  [unwired: 5 in, 1 out]
  n215 = Concatenate Strings("MPP" ("名称（未命名）"), w11) -> (w30:string)
  n216 = Obtain Queue(name (unnamed)=w29, element data type="" ("名称（未命名）")) -> (queue out=w26:refnum<queue>)  [unwired: 3 in, 2 out]
  n217 = property on="窗格" class="Pane"("Origin"=T5 {"Horizontal"=0, "Vertical"=0} ("原点")) -> (error out=w36:errorcluster)  [unwired: 2 in, 1 out]
  n218 = Obtain Queue(name (unnamed)="MT NET Write" ("名称（未命名）"), element data type=T4 {"cmd"=enum."水样测试", "data"=variant} ("簇")) -> (queue out=w7:refnum<queue>)  [unwired: 3 in, 2 out]
  n219 = Obtain Notifier(name (unnamed)=w30, notification data type=FALSE, error in (no error)=w1) -> (notifier out=w6:refnum<notifier>, error out=w3:errorcluster)  [unwired: 1 in, 1 out]
  n220 = Enqueue Element(queue=w26, element="open" ("元素")) -> (queue out=w25:refnum<queue>)  [unwired: 2 in, 2 out]
  n221 = while {
    tunnel: w25 -> [w450]
    stop <- FALSE stop-if-true
    # "断线重连"
    n222 = Wait (ms)(milliseconds to wait=u32 10000 ("等待时间（毫秒）")) -> ()  [unwired: 1 out]
    n223 = global read "断电保存变量.vi" "连接方式"() -> (w451:u16)
    n224 = case shown="1" w451 {
      tunnel: w450 -> [_ w454]
      frame 0, Default {
      }
      frame 1 {
        n225 = case shown="True" "自动断线重连" {
          tunnel: w454 -> [_ w457]
          frame False {
          }
          frame True {
            n226 = global read "多参数全局变量.vi" "MB session in"() -> (w456:refnum<class "MB_Master.lvclass">)
            n227 = property class="MB_Master"(reference=w456) -> ("Properties:Session Valid"=w455:bool)  [unwired: 1 in, 2 out]
            n228 = case shown="False" w455 {
              tunnel: w457 -> [w458 _]
              frame False {
                n229 = Flush Queue(queue=w458) -> (queue out=w460:refnum<queue>)  [unwired: 1 in, 2 out]
                n230 = Enqueue Element(queue=w460, element="open" ("元素")) -> ()  [unwired: 2 in, 3 out]
              }
              frame True {
              }
            }
          }
        }
      }
    }
  }
  n231 = property on="编号" class="Str"("Visible"=w23) -> ()  [unwired: 2 in, 2 out]
  n232 = call "多参数 interface.vi"("error in (no error)"=w3) -> ()  [unwired: 11 in]
  n233 = call "taskqueue ref.vi"() -> ("队列输出"=w4:refnum<queue>)  [unwired: 10 in, 1 out]
  n234 = flat-sequence {
    tunnel: w3 -> [_]
    frame #0 {
      n235 = local read "编号"() -> (w462:string)
      n236 = Equal?(x=w462, y="") -> (x = y?=w464:bool)
      n237 = Select(t="1", s=w464, f=w462) -> (s? t:f=w461:string)
      n238 = call "探头数据读取.vi"("编号"=w461) -> ()  [unwired: 11 in]
    }
  }
  n239 = while {
    tunnel: w25 -> [w467]
    tunnel: w3 -> [_]
    stop <- FALSE stop-if-true
    n240 = Dequeue Element(queue=w467) -> (element=w466:string)  [unwired: 2 in, 3 out]
    n241 = case shown="\"open\"" w466 {
      tunnel: [_ w470 w479] -> _
      frame "假", Default {
      }
      frame "open" {
        n242 = global read "多参数全局变量.vi" "MB session in"() -> (w475:refnum<class "MB_Master.lvclass">)
        n243 = global read "断电保存变量.vi" "VISA资源名称"() -> (w476:refnum<visa-resource-name>)
        n244 = global read "断电保存变量.vi" "Serial Config"() -> (w469:T1)
        n245 = global read "断电保存变量.vi" "连接方式"() -> (w473:u16)
        n246 = call "close MB.vi"("MB session in"=w475) -> ("error out"=w477:errorcluster)  [unwired: 10 in]
        n247 = global read "断电保存变量.vi" "Port"() -> (w471:u16)
        n248 = global read "断电保存变量.vi" "IP"() -> (w472:string)
        n249 = call "open MB.vi"("Port (502)"=w471, "IP Address"=w472, "MODE"=w473, "error in (no error)"=w477, "Serial Config"=w469, "VISA资源名称"=w476) -> ("error out"=w470:errorcluster, "MB session out"=w474:refnum<class "MB_Master.lvclass">)  [unwired: 4 in]
        n250 = global write "多参数全局变量.vi" "MB session in"(w474) -> ()
      }
      frame "close" {
        n251 = global read "多参数全局变量.vi" "MB session in"() -> (w478:refnum<class "MB_Master.lvclass">)
        n252 = call "close MB.vi"("MB session in"=w478) -> ("error out"=w479:errorcluster)  [unwired: 10 in]
      }
    }
  }
  n253 = while {
    tunnel: [w489] -> _
    shift-right: [w483] -> _
    shift-left: _ -> [w487]
    tunnel: w3 -> [w484]
    stop <- FALSE stop-if-true
    n254 = Wait (ms)(milliseconds to wait=u32 1000 ("等待时间（毫秒）")) -> ()  [unwired: 1 out]
    n255 = call <vilib>:"Application Directory.vi"() -> ("Application Directory"=w482:path)
    n256 = Build Path(base path=w482, name or relative path="data\\DCSset.ini" ("名称或相对路径")) -> (appended path=w480:path)
    n257 = File/Directory Info(path=w480, error in=w484) -> (last mod=w483:timestamp, error out=w485:errorcluster)  [unwired: 5 out]
    n258 = Not Equal?(x=w483, y=w487) -> (x != y?=w486:bool)
    n259 = case shown="True" w486 {
      tunnel: [w491 w499] -> w489
      tunnel: w485 -> [w491 w498]
      tunnel: w480 -> [_ w492]
      frame False {
      }
      frame True {
        # "文件发生改变进行更新"
        n260 = call <vilib>:"Open Config Data.vi"("error in (no error)"=w498, "configuration file path"=w492) -> ("error out"=w497:errorcluster, "refnum"=w496:T16)  [unwired: 7 in, 1 out]
        n261 = vi-ref "断电保存变量.vi"() -> (w493:refnum<vi>)
        n262 = call <userlib>:"Read Panel from INI__ogtk.vi"("error in (no error)"=w497, "VI ref"=w493, "refnum"=w496) -> ("error out"=w495:errorcluster, "refnum out"=w494:T16)  [unwired: 7 in]
        n263 = call <vilib>:"Close Config Data.vi"("error in (no error)"=w495, "refnum"=w494) -> ("error out"=w499:errorcluster)  [unwired: 8 in, 1 out]
      }
    }
  }
  n264 = flat-sequence {
    tunnel: w6 -> [w501]
    frame #0 {
      n265 = Obtain Queue(name (unnamed)="MT NET Read" ("名称（未命名）"), element data type=T4 {"cmd"=enum."水样测试", "data"=variant} ("簇")) -> (queue out=w503:refnum<queue>)  [unwired: 3 in, 2 out]
      n266 = call "taskqueue ref.vi"() -> ("队列输出"=w500:refnum<queue>)  [unwired: 10 in, 1 out]
      n267 = while {
        tunnel: w503 -> [w510]
        tunnel: [w508] -> w504
        tunnel: w501 -> [w507]
        tunnel: w500 -> [w506]
        stop <- FALSE stop-if-true
        n268 = Dequeue Element(queue=w510) -> (queue out=w508:refnum<queue>, element=w509:T4)  [unwired: 2 in, 2 out]
        n269 = flat-sequence {
          tunnel: w509 -> [w516]
          tunnel: w507 -> [w513]
          tunnel: w506 -> [w512]
          frame #0 {
            n270 = Unbundle By Name(w516) -> ("cmd"=w515:enum16{"水样测试", "标样核查", "校准状态同步", "停止"}, "data"=w514:variant)
            n271 = case shown="\"标样核查\"" w515 {
              tunnel: w514 -> [w519 _ _ w546]
              tunnel: w513 -> [_ _ w542 _]
              tunnel: w512 -> [w518 _ _ _]
              frame "水样测试", Default {
                n272 = Get Queue Status(queue=w518) -> (# elements in queue=w517:i32)  [unwired: 2 in, 7 out]
                n273 = case shown="0" w517 {
                  tunnel: w519 -> [_ w524]
                  tunnel: w518 -> [_ w521]
                  frame Default {
                  }
                  frame 0 {
                    n274 = global read "断电保存变量.vi" "运行周期"() -> (w526:T14)
                    n275 = Unbundle By Name(w526) -> ("运行模式"=w525:enum16{"维护模式", "常规模式", "应急模式", "质控模式"})
                    n276 = Variant To Data(type="", Variant=w524) -> (data=w522:string)  [unwired: 1 in, 1 out]
                    n277 = case shown="\"常规模式\", Default" w525 {
                      tunnel: ["M" ("数据标记表") w529] -> w520
                      tunnel: w522 -> [_ w528]
                      frame "维护模式" {
                      }
                      frame "常规模式", Default {
                        n278 = case shown="Default" w528 {
                          selector: w528 -> [_ w531]
                          tunnel: ["N" ("数据标记表") w531] -> w529
                          frame Default {
                          }
                          frame "hd" {
                          }
                        }
                      }
                    }
                    n279 = Enqueue Element(queue=w521, element=w520) -> ()  [unwired: 2 in, 3 out]
                  }
                }
              }
              frame "标样核查" {
                n280 = vi-ref "标样核查.vi"() -> (w533:refnum<vi>)
                n281 = property class="VI"(reference=w533) -> ("Name"=w537:string, "Exec.State"=w535:T17)  [unwired: 1 in, 2 out]
                n282 = Open VI Reference(type specifier VI Refnum (for type only)=refnum<vi> refnum, vi path=w537, options=128 ("选项")) -> (vi reference=w538:refnum<vi>)  [unwired: 3 in, 1 out]
                n283 = case shown="\"Idle\"" w535 {
                  tunnel: [w539 w541] -> w534
                  tunnel: w538 -> [w539 w540]
                  frame "Bad", Default {
                  }
                  frame "Idle" {
                    n284 = call-by-ref "开始异步调用"(reference=w540) -> (reference out=w541:refnum<vi>)  [unwired: 13 in, 1 out]
                  }
                }
                n285 = Close Reference(reference=w534) -> ()  [unwired: 1 in, 1 out]
              }
              frame "停止" {
                n286 = Send Notification(notification=TRUE ("通知"), notifier=w542) -> ()  [unwired: 1 in, 2 out]
              }
              frame "校准状态同步" {
                n287 = global read "多参数全局变量.vi" "远程校准运行状态"() -> (w545:T18)
                n288 = Variant To Data(type=w545, Variant=w546) -> (data=w544:T18)  [unwired: 1 in, 1 out]
                n289 = global write "多参数全局变量.vi" "远程校准运行状态"(w544) -> ()
              }
            }
          }
        }
      }
      n290 = call "数据流读取.vi"() -> ()  [unwired: 12 in]
      n291 = call "数据流写入.vi"() -> ()  [unwired: 12 in]
      n292 = Release Queue(queue=w504) -> ()  [unwired: 2 in, 3 out]
    }
  }
  n293 = while {
    tunnel: w36 -> [_]
    tunnel: w6 -> [w550]
    tunnel: w25 -> [w549]
    tunnel: w7 -> [w548]
    tunnel: w4 -> [w547]
    stop <- FALSE stop-if-true
    n294 = event shown="[2] \"量程设置\": Value Change" {
      selector: _ -> [_ _ _ _ _ _ _ _ _ _ _ _ _ _ _ _ _ _ _]
      dyn-events: _ -> [_ _ _ _ _ _ _ _ _ _ _ _ _ _ _ _ _ _ _]
      timeout: _ -> [_ _ _ _ _ _ _ _ _ _ _ _ _ _ _ _ _ _ _]
      tunnel: w550 -> [_ _ _ _ _ _ _ _ _ _ _ _ _ w620 _ _ _ _ _]
      tunnel: w549 -> [_ _ _ _ _ _ _ _ _ _ _ _ _ _ _ _ w632 _ _]
      tunnel: w548 -> [_ _ _ _ _ _ _ _ _ _ _ w595 w603 w618 _ _ _ _ _]
      tunnel: w547 -> [_ _ _ _ _ _ _ _ _ _ _ w591 _ _ _ _ _ _ _]
      event Timeout {
        n295 = event-data() -> ()  [unwired: 1 in, 3 out]
      }
      event "探头设置": Value Change {
        n296 = event-data() -> ()  [unwired: 1 in, 6 out]
        n297 = call "探头启用设置.vi"() -> ()  [unwired: 12 in]
      }
      event "量程设置": Value Change {
        n298 = event-data() -> ()  [unwired: 1 in, 6 out]
        n299 = global read "断电保存变量.vi" "量程参数"() -> (w554:T19)
        n300 = call "量程参数设置对话框.vi"("量程参数"=w554) -> ("布尔"=w552:bool, "量程参数 2"=w553:T19)  [unwired: 9 in]
        n301 = case shown="True" w552 {
          tunnel: w553 -> [_ w555]
          frame False {
          }
          frame True {
            n302 = flat-sequence {
              tunnel: w555 -> [w556]
              frame #0 {
                n303 = global write "断电保存变量.vi" "量程参数"(w556) -> ()
              }
              frame #1 {
                n304 = call "配置文件保存.vi"() -> ()  [unwired: 12 in]
              }
            }
          }
        }
      }
      event "传感器系列号": Value Change {
        n305 = event-data() -> ()  [unwired: 1 in, 6 out]
        n306 = call "系列号查询.vi"() -> ()  [unwired: 12 in]
      }
      event "水样稳定时间", "水样保存组数": Mouse Down {
        n307 = event-data() -> ("CtlRef"=w557:refnum<vi>)  [unwired: 1 in, 7 out]
        n308 = property class="DigNum (strict)"(reference=w557) -> (reference out=w560:refnum<vi>, "Value"=w559:dbl)  [unwired: 1 in, 1 out]
        n309 = call "数字键盘.vi"("OldNumber"=w559) -> ("NewNumber"=w558:dbl)  [unwired: 1 in]
        n310 = property class="DigNum (strict)"(reference=w560, "Val(Sgnl)"=w558) -> ()  [unwired: 1 in, 2 out]
      }
      event "VISA资源名称", "打开modbus", "连接方式", "自动断线重连": Mouse Down {
        n311 = event-data() -> ()  [unwired: 1 in, 6 out]
        n312 = local read "密码锁"() -> (w561:bool)
        n313 = case shown="False" w561 {
          frame False {
            n314 = One Button Dialog(message="当前操作权限不足,请提升权限!!!" ("消息")) -> ()  [unwired: 1 in, 1 out]
          }
          frame True {
          }
        }
      }
      event "IP": Mouse Down {
        n315 = event-data() -> ("CtlRef"=w564:refnum<vi>)  [unwired: 1 in, 7 out]
        n316 = property on="IP" class="Str"() -> ("DisabledEnum"=w563:T6)  [unwired: 2 in, 2 out]
        n317 = case shown="\"Disabled and Grayed Out\"" w563 {
          tunnel: w564 -> [w568 _ _]
          frame "Enabled" {
            n318 = property class="Str"(reference=w568) -> (reference out=w567:refnum<vi>, "Value"=w566:string)  [unwired: 1 in, 1 out]
            n319 = call "字符键盘.vi"("Old String"=w566) -> ("String"=w565:string)  [unwired: 10 in]
            n320 = property class="Str"(reference=w567, "Val(Sgnl)"=w565) -> ()  [unwired: 1 in, 2 out]
          }
          frame "Disabled and Grayed Out" {
            n321 = One Button Dialog(message="关闭连接后才可设置!" ("消息")) -> ()  [unwired: 1 in, 1 out]
          }
          frame "Disabled", Default {
            n322 = One Button Dialog(message="当前操作权限不足,请提升权限!!!" ("消息")) -> ()  [unwired: 1 in, 1 out]
          }
        }
      }
      event "Port": Mouse Down {
        n323 = event-data() -> ("CtlRef"=w572:refnum<vi>)  [unwired: 1 in, 7 out]
        n324 = property on="Port" class="DigNum (strict)"() -> ("DisabledEnum"=w571:T6)  [unwired: 2 in, 2 out]
        n325 = case shown="\"Enabled\"" w571 {
          tunnel: w572 -> [w576 _ _]
          frame "Enabled" {
            n326 = property class="DigNum (strict)"(reference=w576) -> (reference out=w575:refnum<vi>, "Value"=w574:u16)  [unwired: 1 in, 1 out]
            n327 = call "数字键盘.vi"("OldNumber"=w574) -> ("NewNumber"=w573:dbl)  [unwired: 1 in]
            n328 = property class="DigNum (strict)"(reference=w575, "Val(Sgnl)"=w573) -> ()  [unwired: 1 in, 2 out]
          }
          frame "Disabled and Grayed Out" {
            n329 = One Button Dialog(message="关闭连接后才可设置!" ("消息")) -> ()  [unwired: 1 in, 1 out]
          }
          frame "Disabled", Default {
            n330 = One Button Dialog(message="当前操作权限不足,请提升权限!!!" ("消息")) -> ()  [unwired: 1 in, 1 out]
          }
        }
      }
      event "密码锁": Value Change {
        n331 = event-data() -> ("NewVal"=w579:bool)  [unwired: 1 in, 5 out]
        n332 = case shown="True" w579 {
          frame False {
            n333 = global write "多参数全局变量.vi" "权限"(enum16{"一级权限", "二级权限", "三级权限"}."一级权限" ("权限")) -> ()
          }
          frame True {
            n334 = global read "多参数全局变量.vi" "权限密码"() -> (w582:u32[])
            n335 = global read "多参数全局变量.vi" "权限"() -> (w581:enum16{"一级权限", "二级权限", "三级权限", "超级权限"})
            n336 = call "密码权限设置.vi"("权限输入"=w581, "权限密码"=w582) -> ("权限"=w583:enum16{"一级权限", "二级权限", "三级权限", "超级权限"})  [unwired: 9 in]
            n337 = global write "多参数全局变量.vi" "权限"(w583) -> ()
          }
        }
      }
      event "权限等级": Mouse Down {
        n338 = event-data() -> ()  [unwired: 1 in, 8 out]
        n339 = global read "多参数全局变量.vi" "权限密码"() -> (w586:u32[])
        n340 = global read "多参数全局变量.vi" "权限"() -> (w584:enum16{"一级权限", "二级权限", "三级权限", "超级权限"})
        n341 = call "密码权限设置.vi"("权限输入"=w584, "权限密码"=w586) -> ("权限"=w585:enum16{"一级权限", "二级权限", "三级权限", "超级权限"})  [unwired: 9 in]
        n342 = global write "多参数全局变量.vi" "权限"(w585) -> ()
      }
      event "周期设置": Mouse Down {
        n343 = event-data() -> ()  [unwired: 1 in, 6 out]
        n344 = flat-sequence {
          frame #0 {
            n345 = global read "断电保存变量.vi" "定时控制输入"() -> (w588:T12)
            n346 = call "周期设置.vi"("定时控制输入"=w588) -> ("定时控制输出"=w587:T20)  [unwired: 10 in]
            n347 = global write "断电保存变量.vi" "定时控制输入"(w587) -> ()
          }
          frame #1 {
            n348 = call "配置文件保存.vi"() -> ()  [unwired: 12 in]
          }
        }
      }
      event "水样测试": Value Change {
        n349 = event-data() -> ()  [unwired: 1 in, 6 out]
        n350 = Get Queue Status(queue=w591) -> (queue out=w589:refnum<queue>, # elements in queue=w590:i32)  [unwired: 2 in, 6 out]
        n351 = case shown="0" w590 {
          tunnel: w589 -> [_ w597]
          frame Default {
          }
          frame 0 {
            n352 = global read "断电保存变量.vi" "运行周期"() -> (w600:T14)
            n353 = Unbundle By Name(w600) -> ("运行模式"=w599:enum16{"维护模式", "常规模式", "应急模式", "质控模式"})
            n354 = case shown="\"常规模式\", Default" w599 {
              tunnel: ["M" ("数据标记表") w602] -> w596
              tunnel: "hd" ("数据标记表") -> [_ w602]
              frame "维护模式" {
              }
              frame "常规模式", Default {
              }
            }
            n355 = Enqueue Element(queue=w597, element=w596) -> ()  [unwired: 2 in, 3 out]
          }
        }
        n356 = Bundle By Name(cluster=T4 {"cmd"=enum."水样测试", "data"=variant} ("元素"), "data"="hd" ("数据标记表")) -> (w592:T4)
        n357 = Enqueue Element(queue=w595, element=w592) -> ()  [unwired: 2 in, 3 out]
      }
      event "标样核查": Value Change {
        n358 = event-data() -> ()  [unwired: 1 in, 6 out]
        n359 = call "标样核查配置.vi"() -> ("确认输出"=w604:bool)  [unwired: 11 in]
        n360 = case shown="True" w604 {
          tunnel: w603 -> [_ w613]
          frame False {
          }
          frame True {
            n361 = vi-ref "标样核查.vi"() -> (w606:refnum<vi>)
            n362 = property class="VI"(reference=w606) -> ("Name"=w610:string, "Exec.State"=w608:T17)  [unwired: 1 in, 2 out]
            n363 = Enqueue Element(queue=w613, element=T4 {"cmd"=enum."标样核查", "data"=variant} ("元素")) -> ()  [unwired: 2 in, 3 out]
            n364 = Open VI Reference(type specifier VI Refnum (for type only)=refnum<vi> refnum, vi path=w610, options=128 ("选项")) -> (vi reference=w611:refnum<vi>)  [unwired: 3 in, 1 out]
            n365 = case shown="\"Idle\"" w608 {
              tunnel: [w614 w616] -> w607
              tunnel: w611 -> [w614 w615]
              frame "Bad", Default {
              }
              frame "Idle" {
                n366 = call-by-ref "开始异步调用"(reference=w615) -> (reference out=w616:refnum<vi>)  [unwired: 13 in, 1 out]
              }
            }
            n367 = Close Reference(reference=w607) -> ()  [unwired: 1 in, 1 out]
          }
        }
      }
      event "停止": Value Change {
        n368 = event-data() -> ()  [unwired: 1 in, 6 out]
        n369 = Send Notification(notification=TRUE ("通知"), notifier=w620) -> ()  [unwired: 1 in, 2 out]
        n370 = Enqueue Element(queue=w618, element=T4 {"cmd"=enum."停止", "data"=variant} ("元素")) -> ()  [unwired: 2 in, 3 out]
      }
      event "设置": Value Change {
        n371 = event-data() -> ()  [unwired: 1 in, 6 out]
        n372 = property on="窗格" class="Pane"("Origin"=T5 {"Horizontal"=0, "Vertical"=628} ("原点")) -> ()  [unwired: 2 in, 2 out]
        n373 = global write "多参数全局变量.vi" "当前页面"(enum16{"主页面", "参数页面", "校准页面"}."参数页面" ("当前页面")) -> ()
      }
      event "VISA资源名称", "连接方式", "IP", "Port", "自动断线重连", "水样稳定时间", "水样保存组数", "Serial Config": Value Change {
        n374 = event-data() -> ()  [unwired: 1 in, 6 out]
        n375 = flat-sequence {
          frame #0 {
            n376 = global write "断电保存变量.vi" "IP"("IP") -> ()
            n377 = global write "断电保存变量.vi" "Port"("Port") -> ()
            n378 = global write "断电保存变量.vi" "连接方式"("连接方式") -> ()
            n379 = local read "自动断线重连"() -> (w626:bool)
            n380 = global write "断电保存变量.vi" "Serial Config"("Serial Config") -> ()
            n381 = global write "断电保存变量.vi" "水样测试组数"("水样保存组数") -> ()
            n382 = global write "断电保存变量.vi" "水样稳定时间"("水样稳定时间") -> ()
            n383 = global write "断电保存变量.vi" "VISA资源名称"("VISA资源名称") -> ()
            n384 = global write "断电保存变量.vi" "自动断线重连"(w626) -> ()
          }
          frame #1 {
            n385 = call "配置文件保存.vi"() -> ()  [unwired: 12 in]
          }
          frame #2 {
          }
        }
      }
      event "打开modbus": Value Change {
        n386 = event-data() -> ()  [unwired: 1 in, 6 out]
        n387 = global read "多参数全局变量.vi" "MB session in"() -> (w637:refnum<class "MB_Master.lvclass">)
        n388 = Flush Queue(queue=w632) -> (queue out=w631:refnum<queue>)  [unwired: 1 in, 2 out]
        n389 = property class="MB_Master"(reference=w637) -> ("Properties:Session Valid"=w636:bool)  [unwired: 1 in, 2 out]
        n390 = Select(t="close" ("元素"), s=w636, f="open" ("元素")) -> (s? t:f=w633:string)
        n391 = Enqueue Element(queue=w631, element=w633) -> ()  [unwired: 2 in, 3 out]
      }
      event "探头校正返回", "设置页返回": Value Change {
        n392 = event-data() -> ()  [unwired: 1 in, 6 out]
        n393 = property on="窗格" class="Pane"("Origin"=T5 {"Horizontal"=0, "Vertical"=0} ("原点")) -> ()  [unwired: 2 in, 2 out]
        n394 = global write "多参数全局变量.vi" "当前页面"(enum16{"主页面", "参数页面", "校准页面"}."主页面" ("当前页面")) -> ()
      }
      event "探头校正": Value Change {
        n395 = event-data() -> ()  [unwired: 1 in, 6 out]
        n396 = property on="窗格" class="Pane"("Origin"=T5 {"Horizontal"=1656, "Vertical"=0} ("原点")) -> ()  [unwired: 2 in, 2 out]
        n397 = global write "多参数全局变量.vi" "当前页面"(enum16{"主页面", "参数页面", "校准页面"}."校准页面" ("当前页面")) -> ()
        n398 = vi-ref "斯坦道多参数.lvlib:校准UI.vi"() -> (w641:refnum<vi>)
        n399 = property class="VI"(reference=w641) -> (reference out=w643:refnum<vi>, "Exec.State"=w642:T17)  [unwired: 1 in, 1 out]
        n400 = case shown="\"Bad\", Default" w642 {
          tunnel: [w647 w649] -> w645
          tunnel: w643 -> [w647 w648]
          frame "Bad", Default {
          }
          frame "Idle" {
            n401 = invoke class="VI" method="Run VI"(reference=w648, "Wait until done"=FALSE ("结束前等待"), "Auto Dispose Ref"=FALSE ("自动销毁引用")) -> (reference out=w649:refnum<vi>)  [unwired: 2 in, 4 out]
          }
        }
        n402 = invoke on="探头校准子面板" class="SubPnl" method="Remove VI"() -> (error out=w644:errorcluster)  [unwired: 3 in, 2 out]
        n403 = invoke on="探头校准子面板" class="SubPnl" method="Insert VI"(error in=w644, "VI Ref"=w645) -> ()  [unwired: 2 in, 4 out]
      }
    }
  }
